vi "SV Close Work Sheet.vi"(2 "error in (no error)":errorcluster, 3 "Refnum Cluster In":T1) -> (0 "error out":errorcluster, 1 "Refnum Cluster Out":T2)   [LabVIEW 2010]
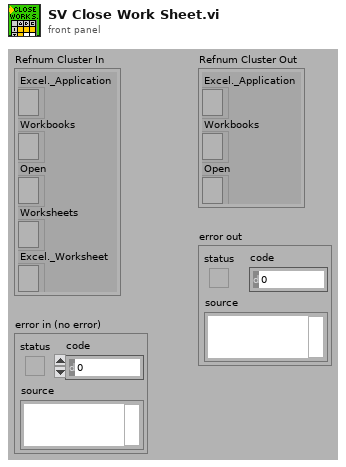
[diagram p1: front panel]
types:
  T1 = cluster{"Excel._Application":refnum<k7>, "Workbooks":refnum<k7>, "Open":refnum<k7>, "Worksheets":refnum<k7>, "Excel._Worksheet":refnum<k7>}
  T2 = cluster{"Excel._Application":refnum<k7>, "Workbooks":refnum<k7>, "Open":refnum<k7>}
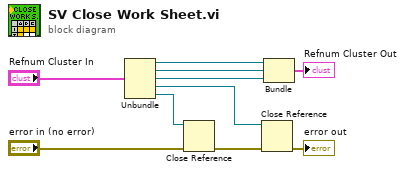
[diagram p0: block diagram]
diagram:
  n1 = Unbundle("Refnum Cluster In") -> ("Excel._Application"=w4:refnum<k7>, "Workbooks"=w3:refnum<k7>, "Open"=w2:refnum<k7>, "Worksheets"=w8:refnum<k7>, "Excel._Worksheet"=w7:refnum<k7>)
  n2 = Close Reference(reference=w7, error in (no error)="error in (no error)") -> (error out=w9:errorcluster)
  n3 = Close Reference(reference=w8, error in (no error)=w9) -> (error out=→"error out":errorcluster)
  n4 = Bundle("Excel._Application"=w4, "Workbooks"=w3, "Open"=w2) -> (→"Refnum Cluster Out":T2)  [unwired: 1 in]
